vi "03询问拆分.vi"(0 "报文":string, 4 "无符号字节数组":u8[](array[numeric]), 10 "功能码":u8) -> (16 "拆分报告":T1, 18 "类别":string)   [LabVIEW 2019, in "MainPage.lvlib" / "MainPage.lvclass"]
uses:
  MainPage.lvclass
panel:
  # "需要前置判断CRC判定\n需要前置判断CRC判定\n需要前置判断CRC判定"
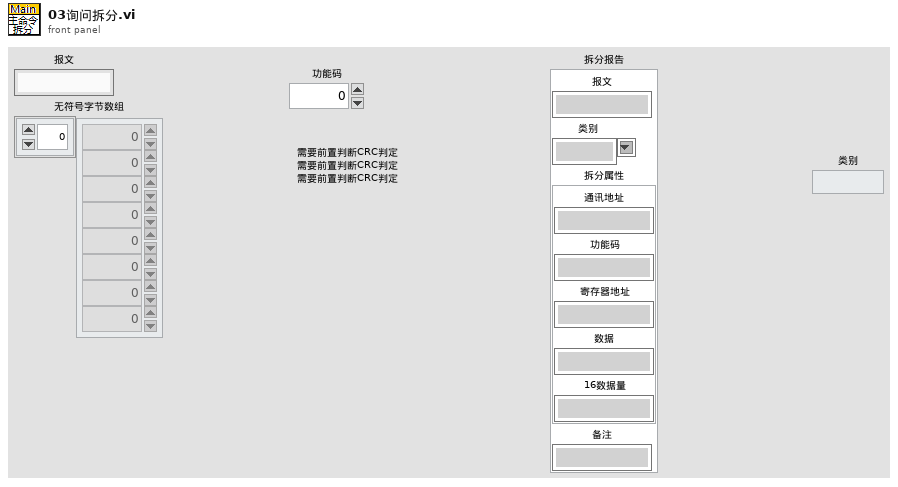
[diagram p1: front panel]
types:
  T1 = cluster{"报文":string, "类别":string, "拆分属性":cluster{"通讯地址":string, "功能码":string, "寄存器地址":string, "数据":string, "16数据量":string}, "备注":string}
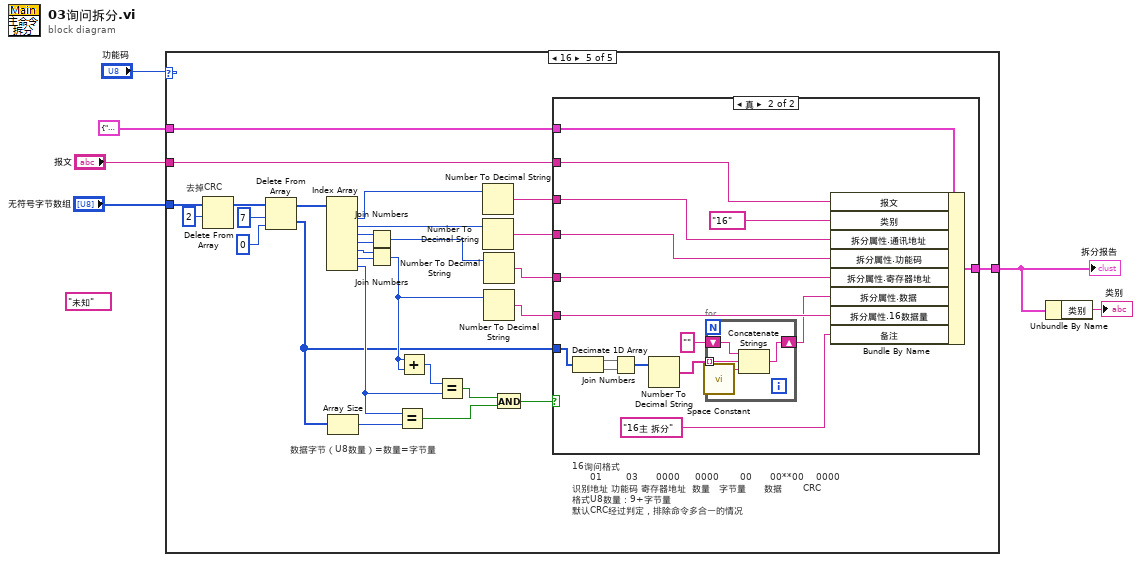
[diagram p0: block diagram]
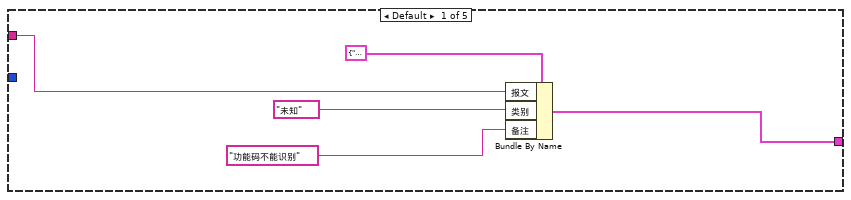
[diagram p2: hidden frame]
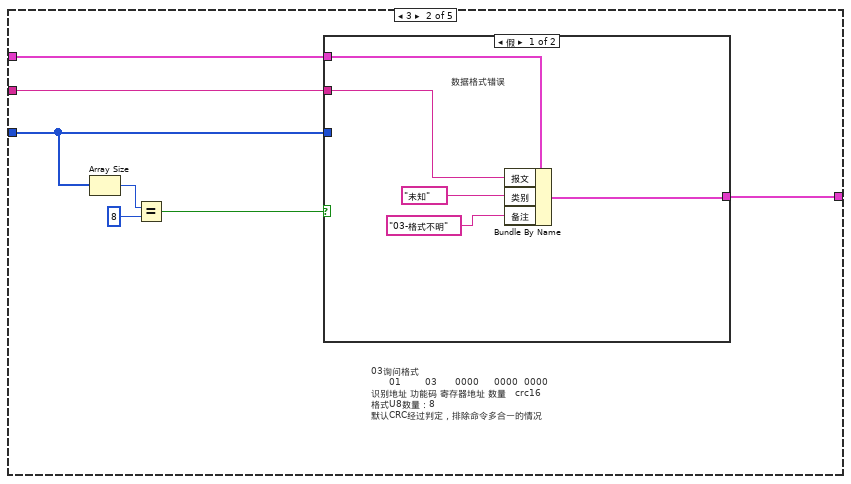
[diagram p3: hidden frame]
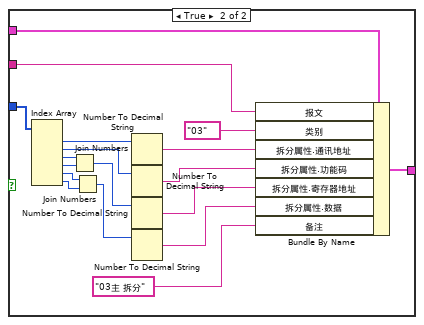
[diagram p4: hidden frame]
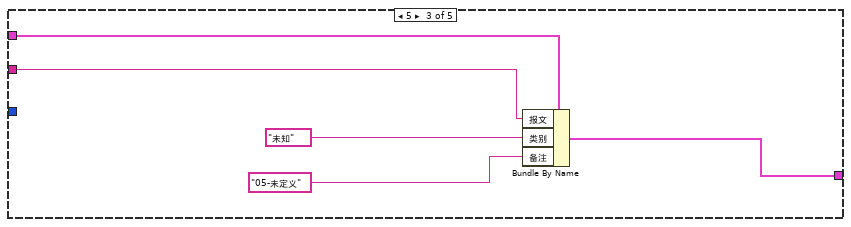
[diagram p5: hidden frame]
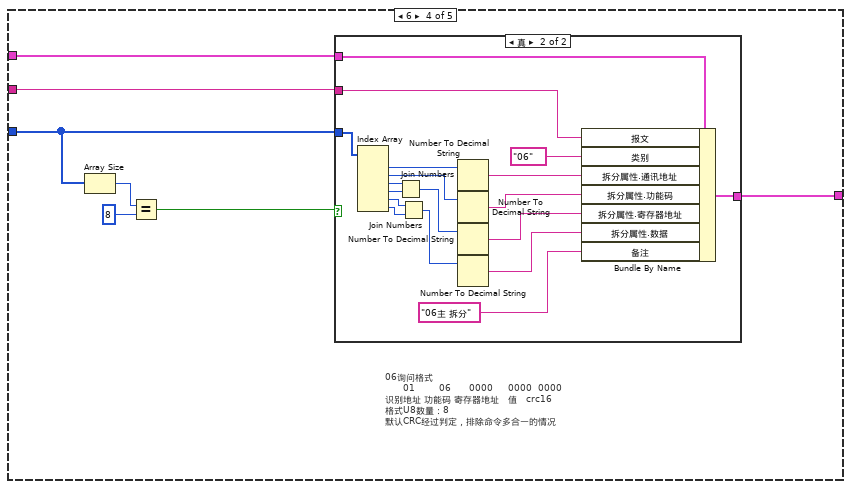
[diagram p6: hidden frame]
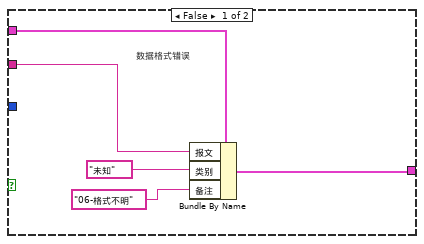
[diagram p7: hidden frame]
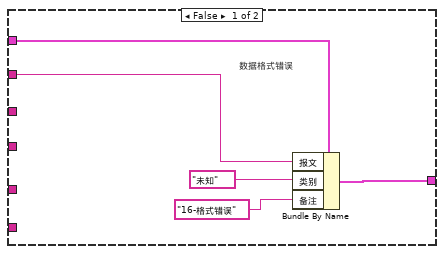
[diagram p8: hidden frame]
diagram:
  (unwired) "未知" ("类别")
  n1 = case shown="16" "功能码" {
    tunnel: "报文" -> [w8 w15 w44 w53 w99]
    tunnel: "无符号字节数组" -> [_ w14 _ w48 w104]
    tunnel: [w7 w13 w46 w51 w96] -> w2
    tunnel: T1 {"报文"="", "类别"="", "拆分属性"={"通讯地址"="", "功能码"="", "寄存器地址"="", "数据"="", "16数据量"=""}, "备注"=""} ("拆分报告") -> [_ w12 w45 w52 w98]
    frame Default {
      n2 = Bundle By Name(cluster=T1 {"报文"="", "类别"="", "拆分属性"={"通讯地址"="", "功能码"="", "寄存器地址"="", "数据"="", "16数据量"=""}, "备注"=""} ("拆分报告"), "报文"=w8, "类别"="未知", "备注"="功能码不能识别") -> (w7:T1)
    }
    frame 3 {
      # "03询问格式\n      01        03      0000     0000  0000\n识别地址 功能码 寄存器地址 数量   crc16\n格式U8数量：8\n默认CRC经过判定，排除命令多合一的情况"
      n3 = Array Size(array=w14) -> (size(s)=w18:i32)
      n4 = Equal?(x=w18, y=8) -> (x = y?=w16:bool)
      n5 = case shown="假" w16 {
        tunnel: w15 -> [w23 w40]
        tunnel: w14 -> [_ w39]
        tunnel: [w20 w41] -> w13
        tunnel: w12 -> [w19 w24]
        frame False {
          # "数据格式错误"
          n6 = Bundle By Name(cluster=w19, "报文"=w23, "类别"="未知", "备注"="03-格式不明") -> (w20:T1)
        }
        frame True {
          n7 = Index Array(array=w39) -> (element #1=w37:u8, element #2=w35:u8, element #3=w33:u8, element #4=w32:u8, element #5=w29:u8, element #6=w28:u8)  [unwired: 6 in]
          n8 = Join Numbers(hi=w33, lo=w32) -> ((hi.lo)=w31:u16)
          n9 = Join Numbers(hi=w29, lo=w28) -> ((hi.lo)=w27:u16)
          n10 = Number To Decimal String(number=w37) -> (decimal integer string=w36:string)  [unwired: 1 in]
          n11 = Number To Decimal String(number=w35) -> (decimal integer string=w34:string)  [unwired: 1 in]
          n12 = Number To Decimal String(number=w31) -> (decimal integer string=w30:string)  [unwired: 1 in]
          n13 = Number To Decimal String(number=w27) -> (decimal integer string=w26:string)  [unwired: 1 in]
          n14 = Bundle By Name(cluster=w24, "报文"=w40, "类别"="03", "拆分属性.通讯地址"=w36, "拆分属性.功能码"=w34, "拆分属性.寄存器地址"=w30, "拆分属性.数据"=w26, "备注"="03主 拆分") -> (w41:T1)
        }
      }
    }
    frame 5 {
      n15 = Bundle By Name(cluster=w45, "报文"=w44, "类别"="未知", "备注"="05-未定义") -> (w46:T1)
    }
    frame 6 {
      # "06询问格式\n      01        06      0000     0000  0000\n识别地址 功能码 寄存器地址   值   crc16\n格式U8数量：8\n默认CRC经过判定，排除命令多合一的情况"
      n16 = Array Size(array=w48) -> (size(s)=w50:i32)
      n17 = Equal?(x=w50, y=8) -> (x = y?=w47:bool)
      n18 = case shown="真" w47 {
        tunnel: w53 -> [w58 w75]
        tunnel: w48 -> [_ w74]
        tunnel: [w55 w76] -> w51
        tunnel: w52 -> [w54 w59]
        frame False {
          # "数据格式错误"
          n19 = Bundle By Name(cluster=w54, "报文"=w58, "类别"="未知", "备注"="06-格式不明") -> (w55:T1)
        }
        frame True {
          n20 = Index Array(array=w74) -> (element #1=w72:u8, element #2=w70:u8, element #3=w68:u8, element #4=w67:u8, element #5=w64:u8, element #6=w63:u8)  [unwired: 6 in]
          n21 = Join Numbers(hi=w68, lo=w67) -> ((hi.lo)=w66:u16)
          n22 = Join Numbers(hi=w64, lo=w63) -> ((hi.lo)=w62:u16)
          n23 = Number To Decimal String(number=w72) -> (decimal integer string=w71:string)  [unwired: 1 in]
          n24 = Number To Decimal String(number=w70) -> (decimal integer string=w69:string)  [unwired: 1 in]
          n25 = Number To Decimal String(number=w66) -> (decimal integer string=w65:string)  [unwired: 1 in]
          n26 = Number To Decimal String(number=w62) -> (decimal integer string=w61:string)  [unwired: 1 in]
          n27 = Bundle By Name(cluster=w59, "报文"=w75, "类别"="06", "拆分属性.通讯地址"=w71, "拆分属性.功能码"=w69, "拆分属性.寄存器地址"=w65, "拆分属性.数据"=w61, "备注"="06主 拆分") -> (w76:T1)
        }
      }
    }
    frame 16 {
      # "数据字节（U8数量）=数量=字节量"
      # "去掉CRC"
      # "16询问格式\n      01        03      0000     0000       00      00**00    0000\n识别地址 功能码 寄存器地址  数量   字节量      数据       CRC\n格式U8数量：9+字节量\n默认CRC经过判定，排除命令多合一的情况"
      n28 = Delete From Array(array=w104, length=2 ("长度")) -> (array with subset deleted=w102:u8[])  [unwired: 1 in, 1 out]
      n29 = Delete From Array(array=w102, length=7 ("长度"), index=0 ("索引")) -> (deleted portion=w77:u8[], array with subset deleted=w97:u8[])
      n30 = Index Array(array=w97) -> (element #1=w87:u8, element #2=w86:u8, element #3=w83:u8, element #4=w82:u8, element #5=w95:u8, element #6=w94:u8, element #7=w91:u8)  [unwired: 7 in]
      n31 = Array Size(array=w77) -> (size(s)=w93:i32)
      n32 = Join Numbers(hi=w83, lo=w82) -> ((hi.lo)=w81:u16)
      n33 = Join Numbers(hi=w95, lo=w94) -> ((hi.lo)=w79:u16)
      n34 = Equal?(x=w91, y=w93) -> (x = y?=w89:bool)
      n35 = Add(x=w79, y=w79) -> (x+y=w92:u16)
      n36 = Equal?(x=w92, y=w91) -> (x = y?=w90:bool)
      n37 = Number To Decimal String(number=w87) -> (decimal integer string=w85:string)  [unwired: 1 in]
      n38 = Number To Decimal String(number=w86) -> (decimal integer string=w84:string)  [unwired: 1 in]
      n39 = Number To Decimal String(number=w81) -> (decimal integer string=w80:string)  [unwired: 1 in]
      n40 = Number To Decimal String(number=w79) -> (decimal integer string=w78:string)  [unwired: 1 in]
      n41 = And(x=w90, y=w89) -> (x .and. y?=w88:bool)
      n42 = case shown="真" w88 {
        tunnel: w99 -> [w109 w124]
        tunnel: [w106 w125] -> w96
        tunnel: w98 -> [w105 w122]
        tunnel: w85 -> [_ w120]
        tunnel: w84 -> [_ w119]
        tunnel: w80 -> [_ w118]
        tunnel: w78 -> [_ w117]
        tunnel: w77 -> [_ w114]
        frame False {
          # "数据格式错误"
          n43 = Bundle By Name(cluster=w105, "报文"=w109, "类别"="未知", "备注"="16-格式错误") -> (w106:T1)
        }
        frame True {
          n44 = Decimate 1D Array(w114) -> (w116:u8[], w115:u8[])
          n45 = Join Numbers(hi=w116, lo=w115) -> ((hi.lo)=w113:u16[])
          n46 = Number To Decimal String(number=w113) -> (decimal integer string=w112:string[])  [unwired: 1 in]
          n47 = for {
            tunnel: w112 -> [w129] mode=indexing
            shift-right: [w127] -> w110
            shift-left: "" -> [w128]
            n48 = call <vilib>:"Space Constant.vi"() -> ("String"=w126:string)
            n49 = Concatenate Strings(w128, w129, w126) -> (w127:string)
          }
          n50 = Bundle By Name(cluster=w122, "报文"=w124, "类别"="16", "拆分属性.通讯地址"=w120, "拆分属性.功能码"=w119, "拆分属性.寄存器地址"=w118, "拆分属性.数据"=w110, "拆分属性.16数据量"=w117, "备注"="16主 拆分") -> (w125:T1)
        }
      }
    }
  }
  "拆分报告" <- w2
  n51 = Unbundle By Name(w2) -> ("类别"=→"类别":string)
